vi "Initialize.vi"(6 "Schedule":string[](array[string]), 8 "error in (no error)":errorcluster, 11 "ID":string) -> (0 "error out":errorcluster, 3 "Minor Frame out":refnum<class "Minor Frame.lvclass">)   [LabVIEW 2020, in "BCI-1553 API.lvlib" / "Minor Frame.lvclass"]
doc: "Generates a Minor Frame object. A Minor Frame has an ID and a Schedule. The ID must be unique to this Minor Frame. The Schedule is an array of strings that determines what Messages (by Message ID) the Minor Frame will be responsible for sending out and what order they will be sent out in. These Messages must be present in the Major Frame that this Minor frame is added to."
uses:
  Minor Frame.lvclass
  Minor Frame.lvclass/Minor Frame.ctl
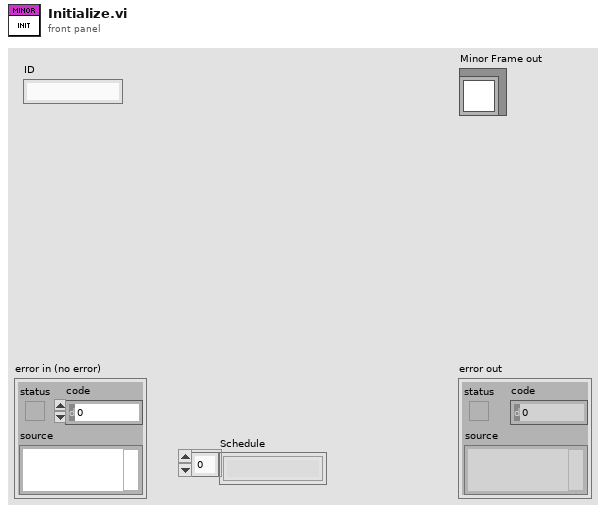
[diagram p1: front panel]
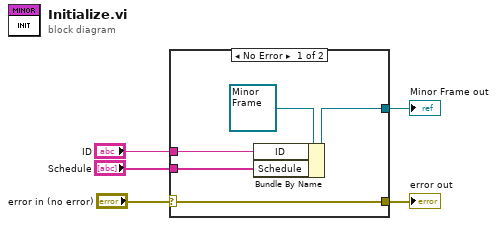
[diagram p0: block diagram]
diagram:
  n1 = case shown="No Error" "error in (no error)" {
    selector: "error in (no error)" -> [w10 w11]
    tunnel: [w10 w11] -> w4
    tunnel: [w8 _] -> w3
    tunnel: "ID" -> [w7 _]
    tunnel: "Schedule" -> [w6 _]
    frame No Error {
      n2 = Bundle By Name(cluster=refnum<class "Minor Frame.lvclass"> refnum ("Minor Frame in"), "ID"=w7, "Schedule"=w6) -> (w8:refnum<class "Minor Frame.lvclass">)
    }
    frame Error {
    }
  }
  "error out" <- w4
  "Minor Frame out" <- w3
